vi "Parse-Clean_Grid.vi"(10 "Tile Array":T1[][](array[typedef])) -> (2 "Cleaned Maze":T1[][](array[typedef]))   [LabVIEW 2020]
doc: "<B>Description:</B> Cleans the Tile array. If there are two lines that are the same, one is removed. If the two line are not the same, then the scan missed a wall line, since that wall didn't actually have a wall in it. (see maze_1 for an example of this). If this is the case, add a new line.\n\n<B>Date:</B> 05/2019\n<B>Author:</B>Luke Jarocki, Choose Movement Consulting, LLC"
uses:
  Controls/TileColor.ctl
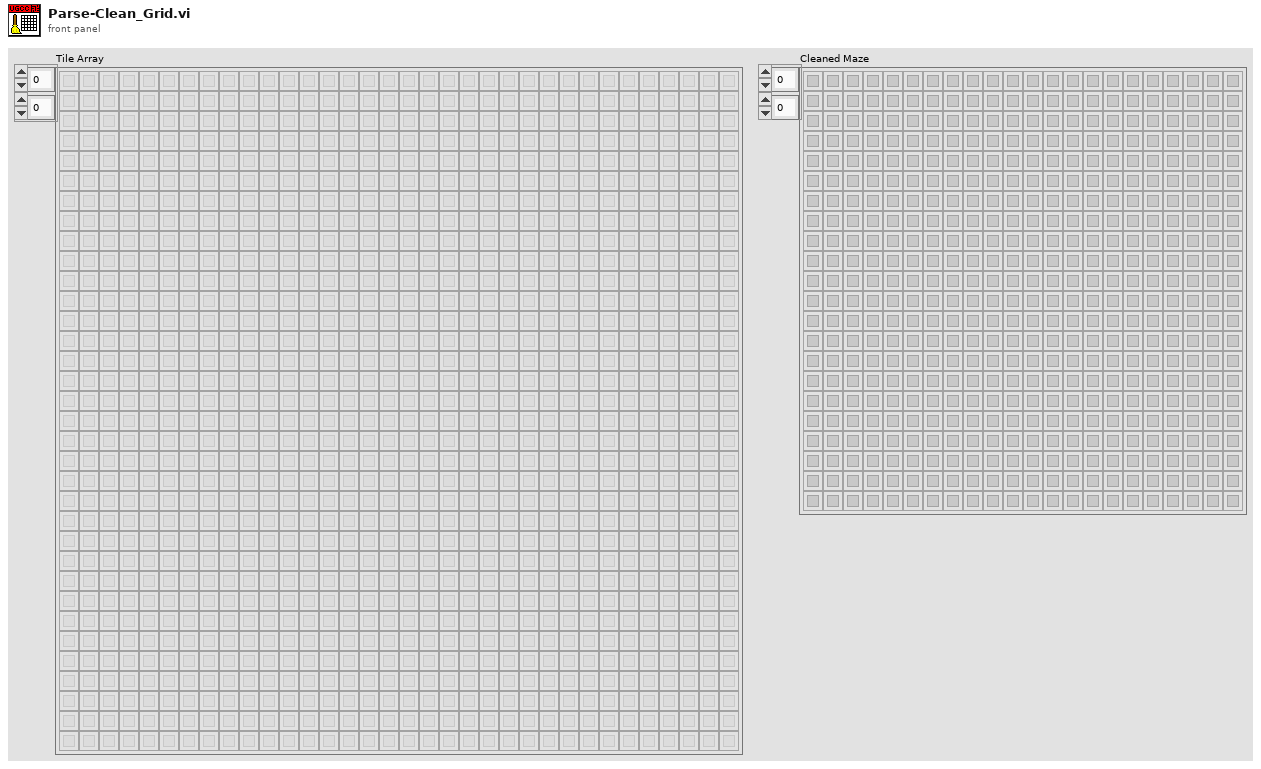
[diagram p1: front panel]
types:
  T1 = typedef "TileColor.ctl" = u16
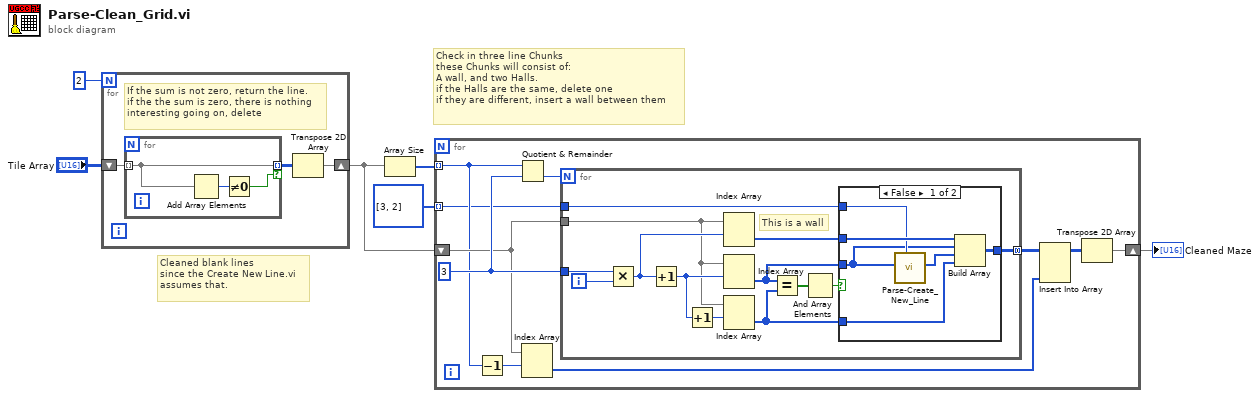
[diagram p0: block diagram]
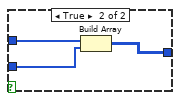
[diagram p2: hidden frame]
diagram:
  # "Check in three line Chunks\nthese Chunks will consist of:\nA wall, and two Halls.\nif the Halls are the same, delete one\nif they are different, insert a wall between them"
  # "Cleaned blank lines\nsince the Create New Line.vi\nassumes that."
  n1 = for {
    N: 2 -> [_]
    shift-right: [w7] -> w4
    shift-left: "Tile Array" -> [w9]
    # "If the sum is not zero, return the line.\nif the the sum is zero, there is nothing\ninteresting going on, delete"
    n2 = for {
      tunnel: w9 -> [w11] mode=indexing
      tunnel: [w11] -> w8 mode=indexing if=w10
      n3 = Add Array Elements(numeric array=w11) -> (sum=w12:T1)
      n4 = Not Equal To 0?(x=w12) -> (x != 0?=w10:bool)
    }
    n5 = Transpose 2D Array(2D array=w8) -> (transposed array=w7:T1[][])
  }
  n6 = Array Size(array=w4) -> (size(s)=w2:i32[])
  n7 = for {
    tunnel: w2 -> [w16] mode=indexing
    shift-right: [w14] -> w3
    shift-left: w4 -> [w18]
    tunnel: i32[] [3, 2] -> [w13] mode=indexing
    w21 = 3 ("y")
    n8 = Decrement(x=w16) -> (x-1=w17:i32)
    n9 = Quotient & Remainder(x=w16, y=w21) -> (floor(x/y)=w22:i32)  [unwired: 1 out]
    n10 = Index Array(array=w18, index (row)=w17) -> (element=w19:T1[])  [unwired: 1 in]
    n11 = for {
      N: w22 -> [_]
      tunnel: w18 -> [w30]
      tunnel: w21 -> [w34]
      tunnel: [w24] -> w20 mode=concatenating
      tunnel: w13 -> [w23]
      i -> [w35]
      # "This is a wall"
      n12 = Multiply(x=w34, y=w35) -> (x*y=w33:i32)
      n13 = Increment(x=w33) -> (x+1=w32:i32)
      n14 = Increment(x=w32) -> (x+1=w31:i32)
      n15 = Index Array(array=w30, index (row)=w33) -> (element=w27:T1[])  [unwired: 1 in]
      n16 = Index Array(array=w30, index (row)=w32) -> (element=w25:T1[])  [unwired: 1 in]
      n17 = Index Array(array=w30, index (row)=w31) -> (element=w26:T1[])  [unwired: 1 in]
      n18 = Equal?(x=w25, y=w26) -> (x = y?=w29:bool[])
      n19 = And Array Elements(Boolean array=w29) -> (logical AND=w28:bool)
      n20 = case shown="False" w28 {
        tunnel: w27 -> [w41 w44]
        tunnel: w26 -> [w38 _]
        tunnel: w25 -> [w39 w43]
        tunnel: [w36 w42] -> w24
        tunnel: w23 -> [w40 _]
        frame False {
          n21 = call "Parse-Create_New_Line.vi"("Interval"=w40, "Existing Row"=w39) -> ("New Row"=w37:T1[])  [unwired: 9 in]
          n22 = Build Array(w41, w39, w37, w38) -> (w36:T1[][])
        }
        frame True {
          n23 = Build Array(w44, w43) -> (w42:T1[][])
        }
      }
    }
    n24 = Insert Into Array(array=w20, new element=w19) -> (w15:T1[][])  [unwired: 2 in]
    n25 = Transpose 2D Array(2D array=w15) -> (transposed array=w14:T1[][])
  }
  "Cleaned Maze" <- w3
